vi "FTW-Request-Reply.vi"(0 "Request":refnum<data-value>, 11 "error in":errorcluster) -> (15 "error out":errorcluster)   [LabVIEW 2015]
doc: "Sends a response message back to the requesting client. This message is attempts to send unconditionally of incoming error. Take caution to wire a sanitized error into this function, because it will be repeated back onto the client. Said another way, an error generated while processing the request will be not only thrown on the request handler, but also on the client as well."
uses:
  json/core/FTW-JSON-Core-Structure.ctl
  error/FTW-ERR-ThrowError.vi
  error/FTW-ERR-CallChain.vi
  string/FTW-STR-ReplaceWhitespace.vi
  string/FTW-STR-Array-Delimit.vi
  error/FTW-ERR-Clear.vi
  regex/FTW-Regex-ReplaceAll.vi
panel:
  # "Inputs"
  # "Outputs"
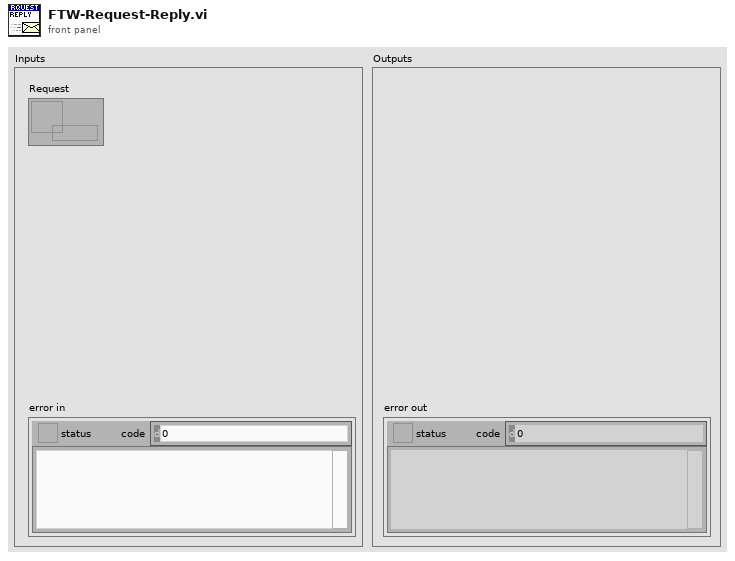
[diagram p1: front panel]
types:
  T1 = typedef "FTW-JSON-Type.ctl" = enum8{"Not Found", "Object", "Array", "String", "Number", "Boolean", "null"}
  T2 = cluster{"Backtrace":i64, "ReplyTimeout":i32, "ReponseIncludesTimestamp":bool, "ReponseIncludesRelativeTimer":bool, "ReponseIncludesException":bool}
  T3 = typedef "FTW-JSON-Core-Structure.ctl" = cluster{"JSON Object":i64, "Encoding Flags":i64, "Decoding Flags":i64}
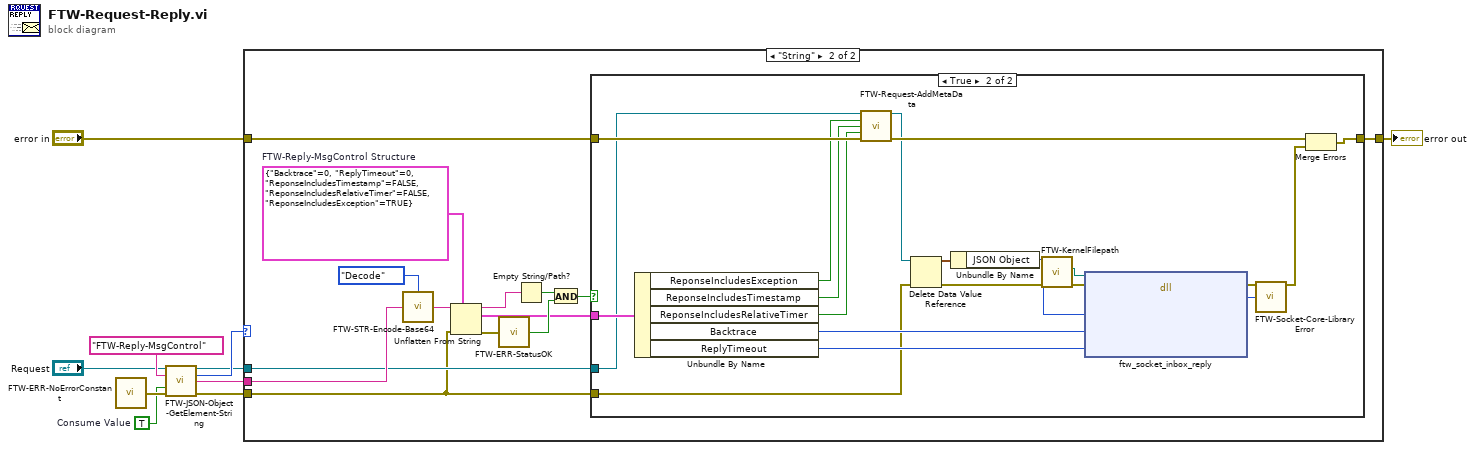
[diagram p0: block diagram]
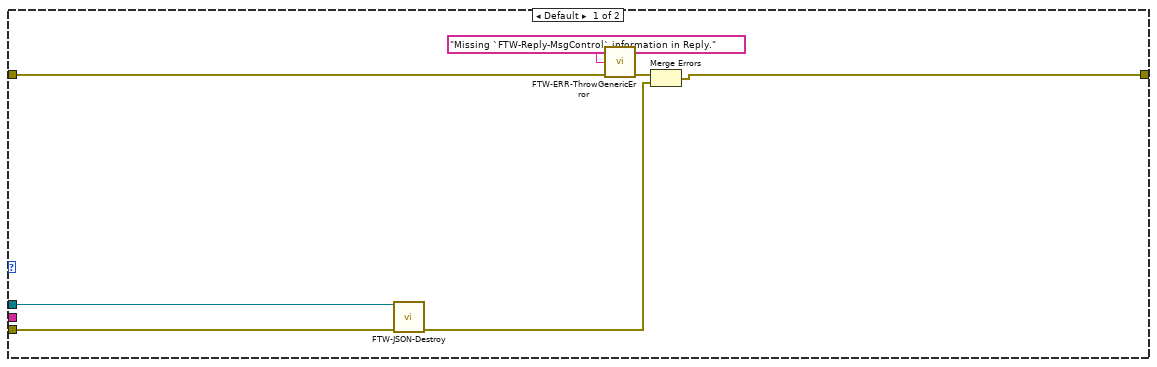
[diagram p2: hidden frame]
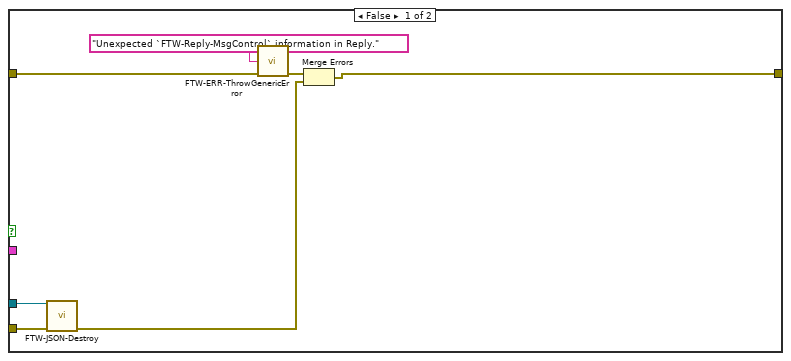
[diagram p3: hidden frame]
diagram:
  w5 = TRUE  # Consume Value
  n1 = call "FTW-ERR-NoErrorConstant.vi"() -> ("no error"=w9:errorcluster)
  n2 = call "FTW-JSON-Object-GetElement-String.vi"("JSON Object"="Request", "Key"="FTW-Reply-MsgControl", "Consume Value"=w5, "error in"=w9) -> ("JSON Object out"=w3:refnum<data-value>, "JSON Element Type"=w4:T1, "Value"=w7:string, "error out"=w6:errorcluster)  [unwired: 8 in]
  n3 = case shown="\"String\"" w4 {
    tunnel: w7 -> [_ w31]
    tunnel: w6 -> [w15 w20]
    tunnel: w3 -> [w16 w21]
    tunnel: "error in" -> [w14 w22]
    tunnel: [w12 w19] -> w1
    frame Default {
      n4 = call "FTW-JSON-Destroy.vi"("JSON Object"=w16, "error in"=w15) -> ("error out"=w11:errorcluster)  [unwired: 13 in]
      n5 = call "FTW-ERR-ThrowGenericError.vi"("Error Message"="Missing `FTW-Reply-MsgControl` information in Reply.", "error in"=w14) -> ("error out"=w13:errorcluster)  [unwired: 13 in]
      n6 = Merge Errors(w13, w11) -> (w12:errorcluster)
    }
    frame "String" {
      w18 = T2 {"Backtrace"=0, "ReplyTimeout"=0, "ReponseIncludesTimestamp"=FALSE, "ReponseIncludesRelativeTimer"=FALSE, "ReponseIncludesException"=TRUE}  # FTW-Reply-MsgControl Structure
      n7 = call "FTW-STR-Encode-Base64.vi"("Input"=w31, "Direction"=enum16{"Encode", "Decode"}."Decode") -> ("Output"=w29:string)
      n8 = Unflatten From String(type=w18, binary string=w29, error in (no error)=w20) -> (rest of the binary string=w28:string, value=w23:T2, error out=w27:errorcluster)  [unwired: 2 in]
      n9 = call "FTW-ERR-StatusOK.vi"("error to check"=w27) -> ("Status OK?"=w25:bool)
      n10 = Empty String/Path?(string/path=w28) -> (empty?=w26:bool)
      n11 = And(x=w26, y=w25) -> (x .and. y?=w24:bool)
      n12 = case shown="True" w24 {
        tunnel: w21 -> [w36 w51]
        tunnel: w22 -> [w37 w56]
        tunnel: [w32 w58] -> w19
        tunnel: w23 -> [_ w57]
        tunnel: w20 -> [w35 w42]
        frame False {
          n13 = call "FTW-JSON-Destroy.vi"("JSON Object"=w36, "error in"=w35) -> ("error out"=w34:errorcluster)  [unwired: 13 in]
          n14 = call "FTW-ERR-ThrowGenericError.vi"("Error Message"="Unexpected `FTW-Reply-MsgControl` information in Reply.", "error in"=w37) -> ("error out"=w33:errorcluster)  [unwired: 13 in]
          n15 = Merge Errors(w33, w34) -> (w32:errorcluster)
        }
        frame True {
          n16 = Unbundle By Name(w57) -> ("ReponseIncludesException"=w50:bool, "ReponseIncludesTimestamp"=w49:bool, "ReponseIncludesRelativeTimer"=w48:bool, "Backtrace"=w47:i64, "ReplyTimeout"=w46:i32)
          n17 = call "FTW-Request-AddMetaData.vi"("Response"=w51, "Include Exception"=w50, "Include Timestamp"=w49, "Include Relative Timer"=w48, "error in"=w56) -> ("Response out"=w45:refnum<data-value>, "error out"=w55:errorcluster)  [unwired: 9 in]
          n18 = Delete Data Value Reference(data value reference=w45, error in=w42) -> (data value=w44:T3, error out=w41:errorcluster)
          n19 = Unbundle By Name(w44) -> ("JSON Object"=w43:i64)
          n20 = call "FTW-KernelFilepath.vi"("error in"=w41) -> ("error out"=w39:errorcluster, "Library Filepath"=w40:path)  [unwired: 8 in, 1 out]
          n21 = dll-call lib="?" fn="ftw_socket_inbox_reply"(path in=w40, error in=w39, "Response"=w43, "Request Backtrace"=w47, "Timeout"=w46) -> (error out=w53:errorcluster, "Return Value"=w54:i64)  [unwired: 4 in, 1 out]
          n22 = call "FTW-Socket-Core-LibraryError.vi"("error in"=w53, "Return Value"=w54) -> ("error out"=w52:errorcluster)  [unwired: 13 in]
          n23 = Merge Errors(w55, w52) -> (w58:errorcluster)
        }
      }
    }
  }
  "error out" <- w1
